vi "GA_mutate.vi"(10 "pop(500*20)":i32[][](array[numeric])) -> (2 "pop(500*20) 2":i32[][](array[numeric]))   [LabVIEW 2018]
uses:
  GA_Global.vi
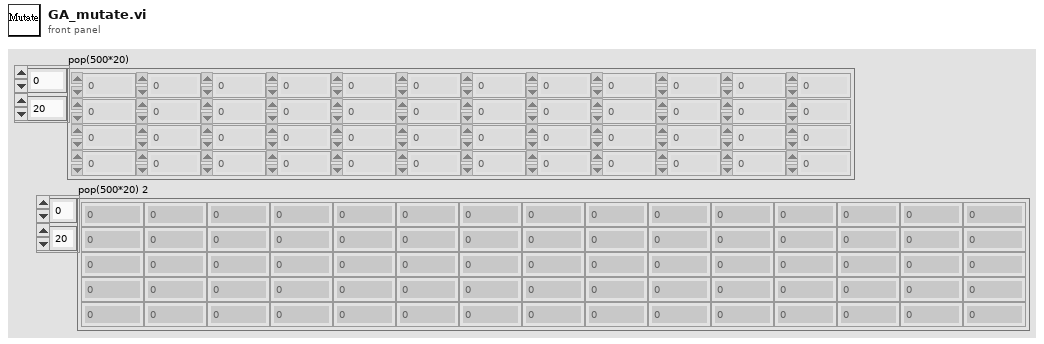
[diagram p1: front panel]
types:
  T1 = typedef "GA_parameter.ctl" = cluster{"N_CITIES":i32, "POP_SIZE":i32, "N_GENERATIONS":i32, "CROSS_RATE":dbl, "MUTATE_RATE":dbl}
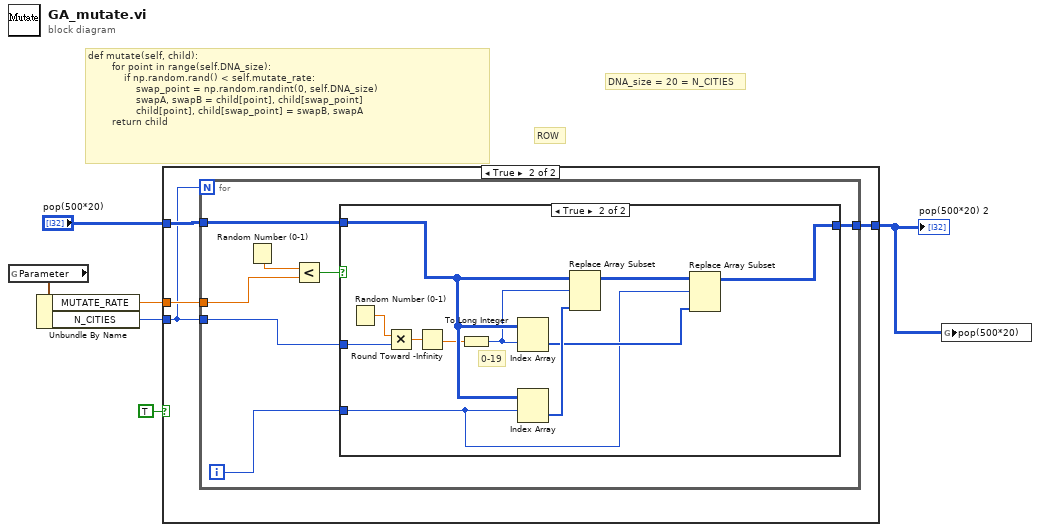
[diagram p0: block diagram]
diagram:
  # "ROW"
  # "DNA_size = 20 = N_CITIES"
  # "def mutate(self, child):\n        for point in range(self.DNA_size):\n            if np.random.rand() < self.mutate_rate:\n                swap_point = np.random.randint(0, self.DNA_size)\n                swapA, swapB = child[point], child[swap_point]\n                child[point], child[swap_point] = swapB, swapA\n        return child"
  n1 = global read "GA_Global.vi" "Parameter"() -> (w5:T1)
  n2 = Unbundle By Name(w5) -> ("MUTATE_RATE"=w4:dbl, "N_CITIES"=w3:i32)
  n3 = case shown="True" TRUE {
    tunnel: "pop(500*20)" -> [w7 w11]
    tunnel: w4 -> [_ w10]
    tunnel: w3 -> [_ w9]
    tunnel: [w7 w8] -> w2
    frame False {
    }
    frame True {
      n4 = for {
        N: w9 -> [_]
        tunnel: w11 -> [w15]
        tunnel: w10 -> [w17]
        tunnel: w9 -> [w16]
        tunnel: [w14] -> w8
        i -> [w12]
        n5 = Random Number (0-1)() -> (number: 0 to 1=w18:dbl)
        n6 = Less?(x=w18, y=w17) -> (x < y?=w13:bool)
        n7 = case shown="True" w13 {
          tunnel: w16 -> [_ w29]
          tunnel: w15 -> [w19 w27]
          tunnel: [w19 w23] -> w14
          tunnel: w12 -> [_ w20]
          frame False {
          }
          frame True {
            # "0-19"
            n8 = Random Number (0-1)() -> (number: 0 to 1=w30:dbl)
            n9 = Multiply(x=w30, y=w29) -> (x*y=w28:dbl)
            n10 = Round Toward -Infinity(1:w28) -> (0:w22:dbl)
            n11 = To Long Integer(number=w22) -> (32bit integer=w21:i32)
            n12 = Index Array(array=w27, index (row)=w21) -> (element=w24:i32[])  [unwired: 1 in]
            n13 = Index Array(array=w27, index (row)=w20) -> (element=w25:i32[])  [unwired: 1 in]
            n14 = Replace Array Subset "Replace Array Subset"(array=w27, new element=w25, index (row)=w21) -> (w26:i32[][])  [unwired: 1 in]
            n15 = Replace Array Subset "Replace Array Subset"(array=w26, new element=w24, index (row)=w20) -> (w23:i32[][])  [unwired: 1 in]
          }
        }
      }
    }
  }
  "pop(500*20) 2" <- w2
  n16 = global write "GA_Global.vi" "pop(500*20)"(w2) -> ()
